vi "main.vi"() -> ()   [LabVIEW 2022 SP3]
uses:
  <vilib>/DAQmx/read.llb/DAQmx Read (Analog 1D DBL NChan 1Samp).vi
  <vilib>/DAQmx/write.llb/DAQmx Write (Digital Bool 1Line 1Point).vi
  <vilib>/DAQmx/read.llb/DAQmx Read (Digital Bool 1Line 1Point).vi
  <vilib>/DAQmx/create/channels.llb/DAQmx Create Channel (DI-Digital Input).vi
  <vilib>/DAQmx/miscellaneous.llb/DAQmx Fill In Error Info.vi
  <vilib>/DAQmx/create/channels.llb/DAQmx Create Channel (AI-Voltage-Basic).vi
  <vilib>/DAQmx/create/channels.llb/DAQmx Create Channel (DO-Digital Output).vi
panel:
  out "Solar":dbl
  out "IR":dbl
  in  "data 6":bool
  in  "data 5":bool
  in  "data 4":bool
  in  "data 3":bool
  in  "stop":bool
  out "data 2":bool
  out "data":bool
  out "line2":i16
  out "line1":i16
  out "String":string
  in  "stop (F) 2":bool caption="stop (F)"
  out "Square 2":dynamicdata(graph) caption="Square"
  in  "Frequency 2":dbl=50.0 caption="Frequency"
  in  "Offset 2":dbl=2.5 caption="Offset"
  in  "Amplitude 2":dbl=2.5 caption="Amplitude"
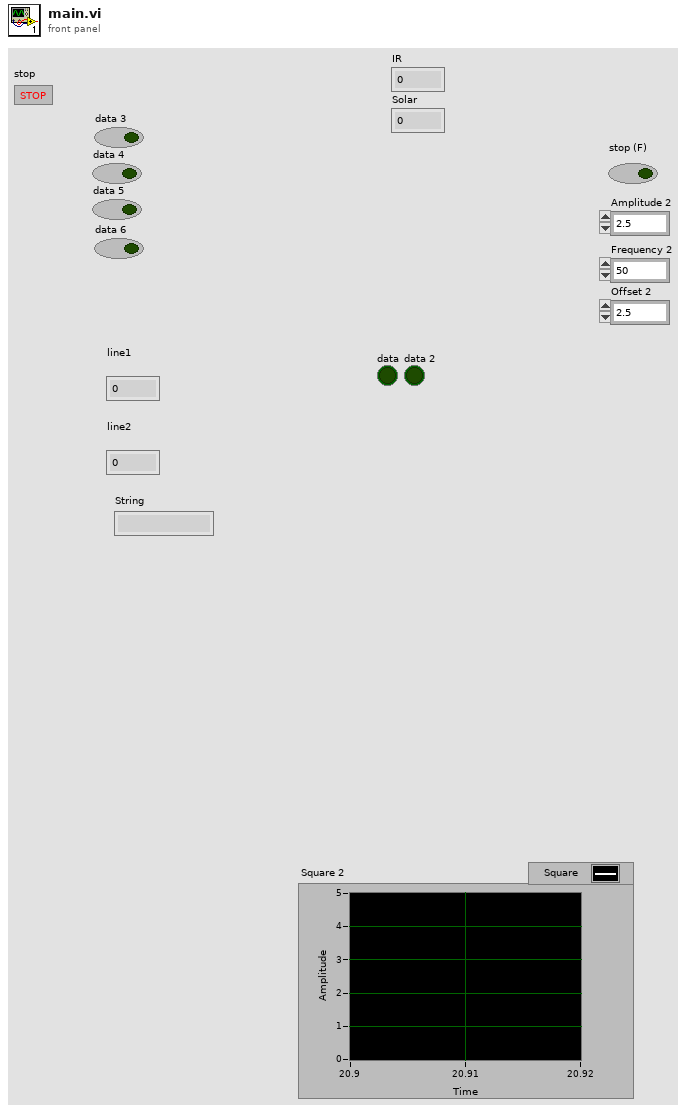
[diagram p1: front panel]
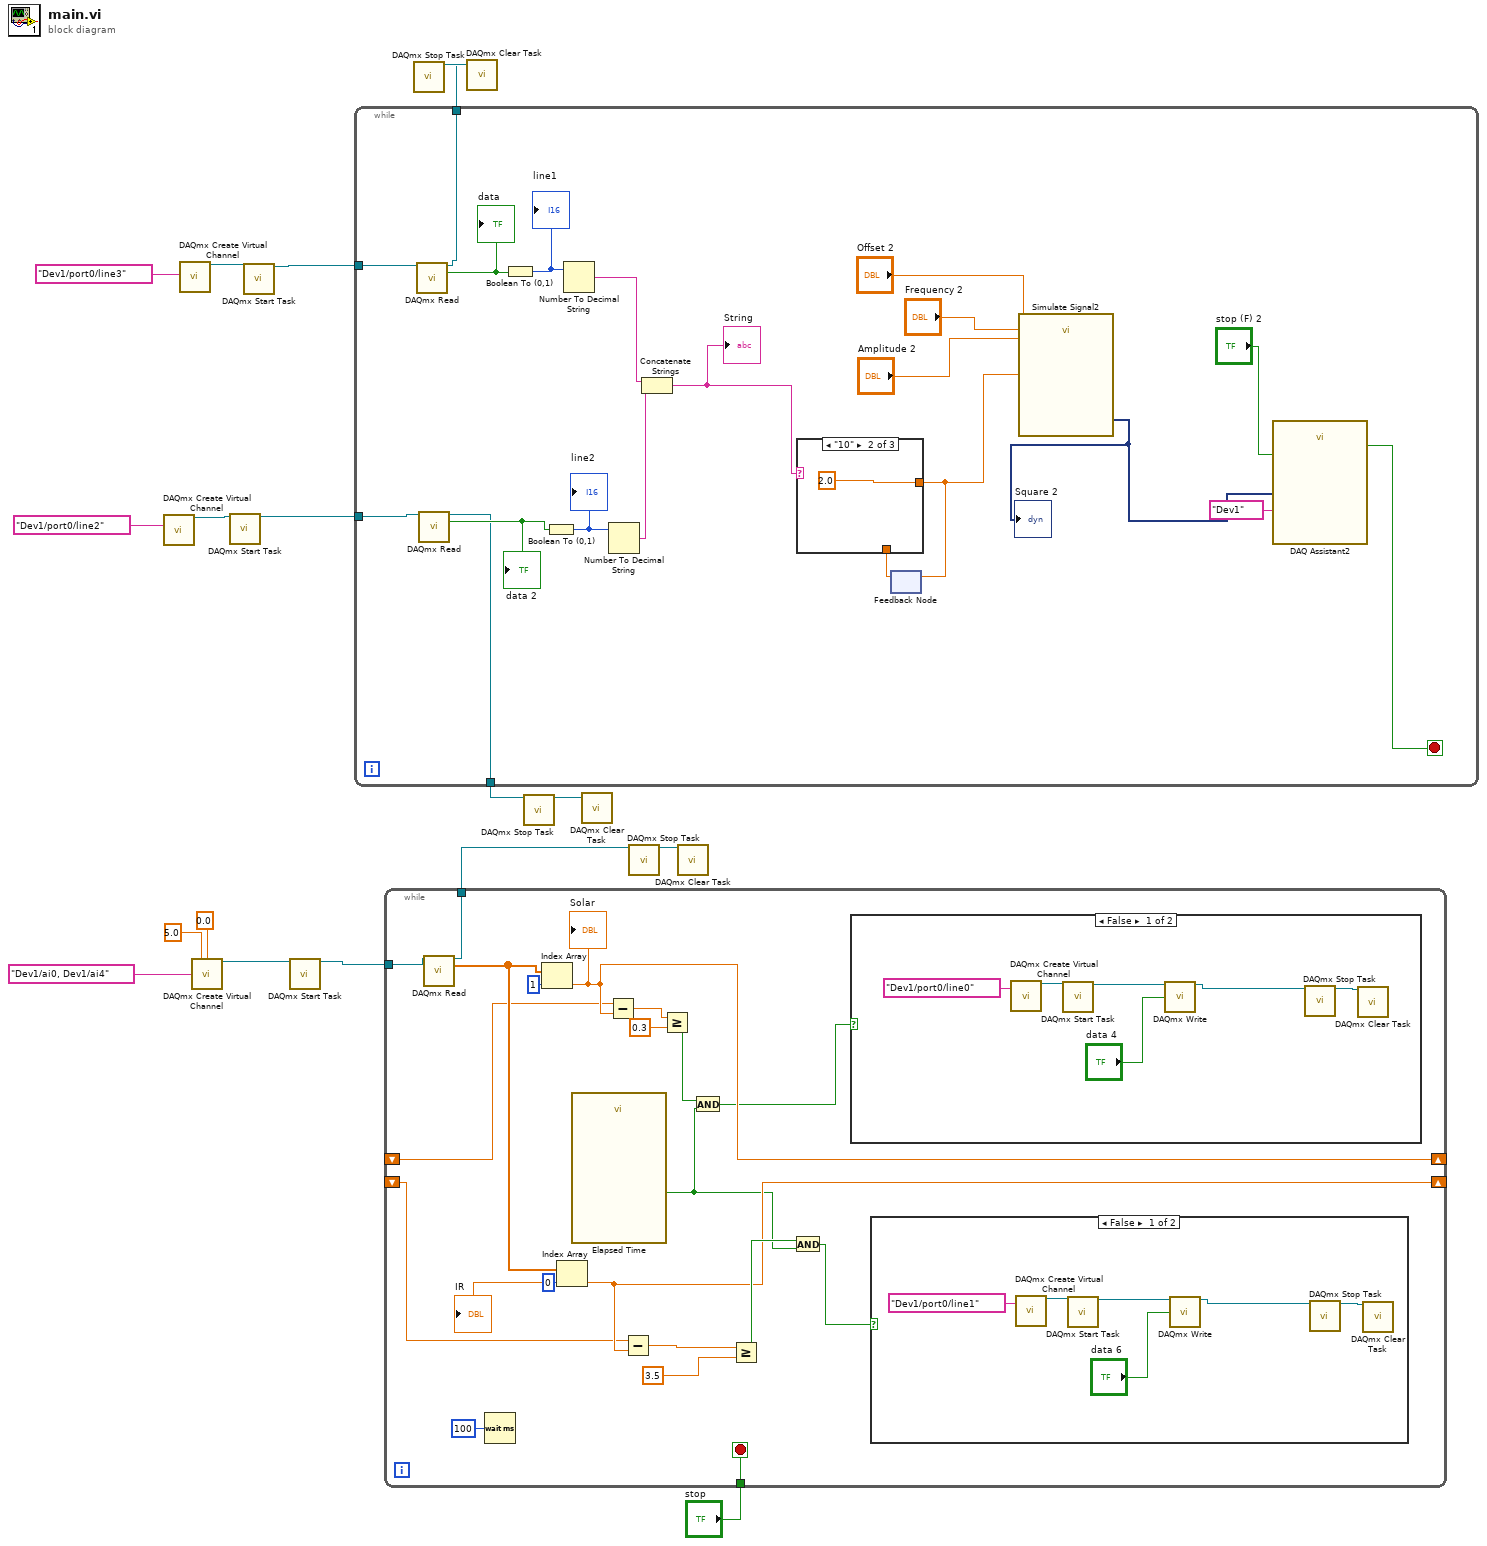
[diagram p0: block diagram]
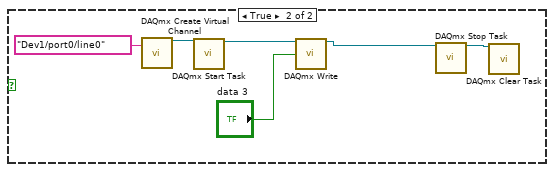
[diagram p2: hidden frame]
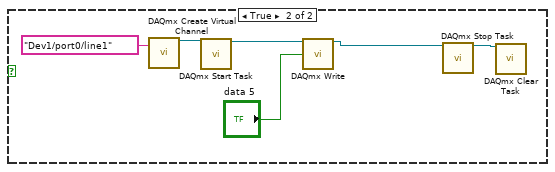
[diagram p3: hidden frame]
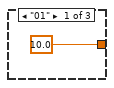
[diagram p4: hidden frame]
diagram:
  n1 = call-poly <vilib>:"DAQmx Create Virtual Channel.vi"("lines"=tag "Dev1/port0/line2") -> ("task out"=w15:refnum<k21>)  [unwired: 13 in, 1 out]
  n2 = call-poly <vilib>:"DAQmx Create Virtual Channel.vi"("lines"=tag "Dev1/port0/line3") -> ("task out"=w18:refnum<k21>)  [unwired: 13 in, 1 out]
  n3 = call-poly <vilib>:"DAQmx Create Virtual Channel.vi"("maximum value"=5.0, "minimum value"=0.0, "physical channels"=tag "Dev1/ai0, Dev1/ai4") -> ("task out"=w4:refnum<k21>)  [unwired: 11 in, 1 out]
  n4 = call <vilib>:"DAQmx Start Task.vi"("task/channels in"=w15) -> ("task out"=w13:refnum<k21>)  [unwired: 13 in, 1 out]
  n5 = call <vilib>:"DAQmx Start Task.vi"("task/channels in"=w18) -> ("task out"=w16:refnum<k21>)  [unwired: 13 in, 1 out]
  n6 = call <vilib>:"DAQmx Start Task.vi"("task/channels in"=w4) -> ("task out"=w6:refnum<k21>)  [unwired: 13 in, 1 out]
  n7 = while {
    tunnel: w16 -> [w30]
    tunnel: w13 -> [w32]
    tunnel: [w31] -> w11
    tunnel: [w29] -> w9
    stop <- w28 stop-if-true
    n8 = call-poly <vilib>:"DAQmx Read.vi"("task/channels in"=w30) -> ("task out"=w31:refnum<k21>, "data"=w37:bool)  [unwired: 12 in, 1 out]
    "data" <- w37
    n9 = call-poly <vilib>:"DAQmx Read.vi"("task/channels in"=w32) -> ("task out"=w29:refnum<k21>, "data"=w38:bool)  [unwired: 12 in, 1 out]
    "data 2" <- w38
    n10 = Boolean To (0,1)(Boolean=w37) -> (0, 1=w36:i16)
    "line1" <- w36
    n11 = Boolean To (0,1)(Boolean=w38) -> (0, 1=w35:i16)
    "line2" <- w35
    n12 = Number To Decimal String(number=w36) -> (decimal integer string=w34:string)  [unwired: 1 in]
    n13 = Number To Decimal String(number=w35) -> (decimal integer string=w33:string)  [unwired: 1 in]
    n14 = Concatenate Strings(w34, w33) -> (w21:string)
    "String" <- w21
    n15 = feedback #1() -> (w19:dbl)  [unwired: 1 in]
    n16 = case shown="\"10\"" w21 {
      tunnel: [10.0 ("Duty Cycle (%)") 2.0 ("Duty Cycle (%)") w41] -> w20
      tunnel: w19 -> [_ _ w41]
      frame "01" {
      }
      frame "10" {
      }
      frame Default {
      }
    }
    n17 = feedback-in #1(w20) -> ()
    n18 = call "Simulate Signal2"("Offset"="Offset 2", "Duty Cycle (%)"=w20, "Frequency"="Frequency 2", "Amplitude"="Amplitude 2") -> ("Square"=w23:dynamicdata)  [unwired: 10 in, 1 out]
    "Square 2" <- w23
    n19 = call "DAQ Assistant2"("data"=w23, "stop (F)"="stop (F) 2", "device name"=tag "Dev1") -> ("stopped"=w28:bool)  [unwired: 14 in, 2 out]
  }
  n20 = while {
    tunnel: "stop" -> [w61]
    shift-right: [w49] -> _
    shift-left: _ -> [w42]
    tunnel: w6 -> [w56]
    shift-right: [w48] -> _
    shift-left: _ -> [w47]
    tunnel: [w43] -> w3
    stop <- w61 stop-if-true
    n21 = call-poly <vilib>:"DAQmx Read.vi"("task/channels in"=w56) -> ("task out"=w43:refnum<k21>, "data"=w50:dbl[])  [unwired: 12 in, 1 out]
    n22 = Wait (ms)(milliseconds to wait=u32 100) -> ()  [unwired: 1 out]
    n23 = Index Array(array=w50, index=1) -> (element=w49:dbl)
    "Solar" <- w49
    n24 = Index Array(array=w50, index=0) -> (element=w48:dbl)
    "IR" <- w48
    n25 = call "Elapsed Time"() -> ("Time has Elapsed"=w46:bool)  [unwired: 12 in, 7 out]
    n26 = Subtract(x=w42, y=w49) -> (x-y=w59:dbl)
    n27 = Subtract(x=w47, y=w48) -> (x-y=w53:dbl)
    n28 = Greater Or Equal?(x=w59, y=0.3) -> (x >= y?=w60:bool)
    n29 = And(x=w60, y=w46) -> (x .and. y?=w44:bool)
    n30 = Greater Or Equal?(x=w53, y=3.5) -> (x >= y?=w54:bool)
    n31 = And(x=w54, y=w46) -> (x .and. y?=w45:bool)
    n32 = case shown="False" w44 {
      frame False {
        n33 = call-poly <vilib>:"DAQmx Create Virtual Channel.vi"("lines"=tag "Dev1/port0/line0") -> ("task out"=w64:refnum<k21>)  [unwired: 13 in, 1 out]
        n34 = call <vilib>:"DAQmx Start Task.vi"("task/channels in"=w64) -> ("task out"=w65:refnum<k21>)  [unwired: 13 in, 1 out]
        n35 = call-poly <vilib>:"DAQmx Write.vi"("task/channels in"=w65, "data"="data 4") -> ("task out"=w62:refnum<k21>)  [unwired: 11 in, 2 out]
        n36 = call <vilib>:"DAQmx Stop Task.vi"("task/channels in"=w62) -> ("task out"=w66:refnum<k21>)  [unwired: 13 in, 1 out]
        n37 = call <vilib>:"DAQmx Clear Task.vi"("task in"=w66) -> ()  [unwired: 14 in, 1 out]
      }
      frame True {
        n38 = call-poly <vilib>:"DAQmx Create Virtual Channel.vi"("lines"=tag "Dev1/port0/line0") -> ("task out"=w70:refnum<k21>)  [unwired: 13 in, 1 out]
        n39 = call <vilib>:"DAQmx Start Task.vi"("task/channels in"=w70) -> ("task out"=w71:refnum<k21>)  [unwired: 13 in, 1 out]
        n40 = call-poly <vilib>:"DAQmx Write.vi"("task/channels in"=w71, "data"="data 3") -> ("task out"=w68:refnum<k21>)  [unwired: 11 in, 2 out]
        n41 = call <vilib>:"DAQmx Stop Task.vi"("task/channels in"=w68) -> ("task out"=w72:refnum<k21>)  [unwired: 13 in, 1 out]
        n42 = call <vilib>:"DAQmx Clear Task.vi"("task in"=w72) -> ()  [unwired: 14 in, 1 out]
      }
    }
    n43 = case shown="False" w45 {
      frame False {
        n44 = call-poly <vilib>:"DAQmx Create Virtual Channel.vi"("lines"=tag "Dev1/port0/line1") -> ("task out"=w76:refnum<k21>)  [unwired: 13 in, 1 out]
        n45 = call <vilib>:"DAQmx Start Task.vi"("task/channels in"=w76) -> ("task out"=w77:refnum<k21>)  [unwired: 13 in, 1 out]
        n46 = call-poly <vilib>:"DAQmx Write.vi"("task/channels in"=w77, "data"="data 6") -> ("task out"=w74:refnum<k21>)  [unwired: 11 in, 2 out]
        n47 = call <vilib>:"DAQmx Stop Task.vi"("task/channels in"=w74) -> ("task out"=w78:refnum<k21>)  [unwired: 13 in, 1 out]
        n48 = call <vilib>:"DAQmx Clear Task.vi"("task in"=w78) -> ()  [unwired: 14 in, 1 out]
      }
      frame True {
        n49 = call-poly <vilib>:"DAQmx Create Virtual Channel.vi"("lines"=tag "Dev1/port0/line1") -> ("task out"=w82:refnum<k21>)  [unwired: 13 in, 1 out]
        n50 = call <vilib>:"DAQmx Start Task.vi"("task/channels in"=w82) -> ("task out"=w83:refnum<k21>)  [unwired: 13 in, 1 out]
        n51 = call-poly <vilib>:"DAQmx Write.vi"("task/channels in"=w83, "data"="data 5") -> ("task out"=w80:refnum<k21>)  [unwired: 11 in, 2 out]
        n52 = call <vilib>:"DAQmx Stop Task.vi"("task/channels in"=w80) -> ("task out"=w84:refnum<k21>)  [unwired: 13 in, 1 out]
        n53 = call <vilib>:"DAQmx Clear Task.vi"("task in"=w84) -> ()  [unwired: 14 in, 1 out]
      }
    }
  }
  n54 = call <vilib>:"DAQmx Stop Task.vi"("task/channels in"=w11) -> ("task out"=w12:refnum<k21>)  [unwired: 13 in, 1 out]
  n55 = call <vilib>:"DAQmx Clear Task.vi"("task in"=w12) -> ()  [unwired: 14 in, 1 out]
  n56 = call <vilib>:"DAQmx Stop Task.vi"("task/channels in"=w9) -> ("task out"=w10:refnum<k21>)  [unwired: 13 in, 1 out]
  n57 = call <vilib>:"DAQmx Clear Task.vi"("task in"=w10) -> ()  [unwired: 14 in, 1 out]
  n58 = call <vilib>:"DAQmx Stop Task.vi"("task/channels in"=w3) -> ("task out"=w5:refnum<k21>)  [unwired: 13 in, 1 out]
  n59 = call <vilib>:"DAQmx Clear Task.vi"("task in"=w5) -> ()  [unwired: 14 in, 1 out]
